vi "PH_Sixpack.set Status.vi"(0 "VI in":refnum<vi>, 2 "Status":T1, 5 "error in (no error)":errorcluster) -> (14 "VI out":refnum<vi>, 19 "error out":errorcluster)   [LabVIEW 2014, in "PH_Sixpack.lvlib"]
doc: "This VI sets the internal status."
uses:
  PH_Sixpack.lvlib
  PH_Sixpack.Status.ctl
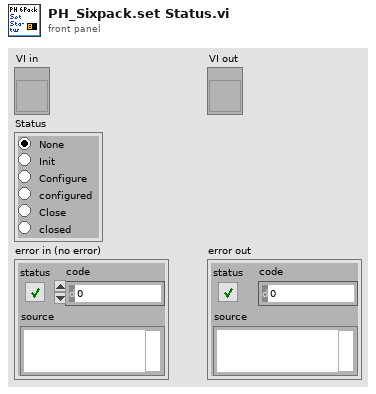
[diagram p1: front panel]
types:
  T1 = typedef "PH_Sixpack.lvlib/PH_Sixpack.Status.ctl" = enum32{"None", "Init", "Configure", "configured", "Close", "closed"}
  T2 = typedef "PH_Sixpack.lvlib/PH_Sixpack.i attribute.ctl" = cluster{"Information":cluster{"SixPack ID(0)":u16, "BaudRate(19200)":u16, "COM Port":enum32{"COM1", "COM2", "COM3", "COM4", "COM5", "COM6", "COM7", "COM8", "COM9"}, "HANDLE":i32}, "Serial Number":dbl, "Firmwareversion":dbl, "Axes":T3[], "Status":T1, "Axis to do a RefSearch":i32, "GUI Refs":cluster{"Information":refnum<vi>, "Serial Number":refnum<vi>, "Firmwareversion":refnum<vi>, "Status":refnum<vi>, "Axis to do a RefSearch":refnum<vi>, "Axes Configuration (Sixpack)":refnum<vi>, "Inputs":refnum<vi>, "PeriodicInterval [ms]":refnum<vi>}, "Constructor finished":bool, "Ignore Error":bool}
  T3 = typedef "PH_Sixpack.lvlib/PH_Sixpack.Axis Cluster.ctl" = cluster{"Config":T4, "To set?":cluster{"VmaxAmax":bool, "I max":bool, "VStartVminDivi":bool, "Ref Search Parameter":bool, "Stopswitch Limits":bool, "Axis Parameter":bool, "I Control":bool}}
  T4 = typedef "PH_Sixpack.lvlib/PH_Sixpack.Axis Configuration.ctl" = cluster{"VmaxAmax":T5, "I max (50%)":T6, "VStartVminDivi":T7, "Ref Search Parameter":T8, "Stopswitch Limits":T9, "Axis Parameter":T10, "I Control":T13}
  T5 = typedef "Sixpack - Driver.lvlib/VmaxAmax.ctl" = cluster{"VMax(511)":u16, "AMax(128)":u16}
  T6 = typedef "Sixpack - Driver.lvlib/PeakCurrent.ctl" = dbl
  T7 = typedef "Sixpack - Driver.lvlib/VStartVmin.ctl" = cluster{"VStart(5)":u16, "Vmin(4)":u16, "Div i (2)":enum8{"0", "1", "2", "3"}}
  T8 = typedef "Sixpack - Driver.lvlib/Ref Search Parameter.ctl" = cluster{"VRefMax(100)":u16, "DebouncingTime (22ms)":u8}
  T9 = typedef "Sixpack - Driver.lvlib/Stopswitch Limits.ctl" = cluster{"MinLeft(0)":u16, "MaxRight(1023)":u16}
  T10 = typedef "Sixpack - Driver.lvlib/Motor Parameter.ctl" = cluster{"Poslimit (6400)":u32, "P5 Bits":T11, "P6 Bits":T12}
  T11 = typedef "Sixpack - Driver.lvlib/MotorParameter_P5.ctl" = cluster{"MT_PI":bool, "MT_ROTARY":bool, "MT_AUTONULLCMD":bool, "MT_TESTNULL":bool, "MT_NULLLEFT":bool, "MT_NULLCENTRE":bool, "MT_STOPNULL":bool, "MT_FILTERSWITCH":bool}
  T12 = typedef "Sixpack - Driver.lvlib/MotorParameter_P6.ctl" = cluster{"MT_OPTIMIZEWAY":bool, "MT_FASTREF":bool, "MT_MECHREF":bool, "MT_DELAYTESTNULL":bool, "MT_STOPSOFT":bool, "MT_STOPNOREF":bool, "MT_NULLPOSITIVE":bool, "MUT_STOPFULSTEPS":bool}
  T13 = typedef "Sixpack - Driver.lvlib/Current Control.ctl" = cluster{"PowerDownDelay (500)":u16, "PowerDown (0%)":T14, "Standing (50%)":T14, "Running (75%)":T14, "Accelerating (100%)":T14}
  T14 = typedef "Sixpack - Driver.lvlib/Current.ctl" = enum8{"100%", "75%", "50%", "38%", "25%", "19%", "13%", "9%", "0%"}
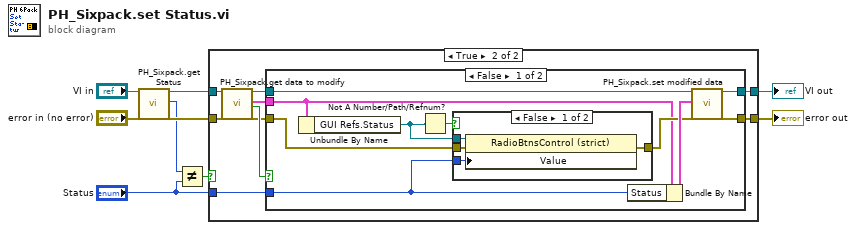
[diagram p0: block diagram]
diagram:
  n1 = call "PH_Sixpack.get Status.vi"("VI in"="VI in", "error in (no error)"="error in (no error)") -> ("VI out"=w6:refnum<vi>, "Status"=w5:T1, "error out"=w7:errorcluster)  [unwired: 14 in, 1 out]
  n2 = Not Equal?(x=w5, y="Status") -> (x != y?=w3:bool)
  n3 = case shown="True" w3 {
    tunnel: [w10 w20] -> w9
    tunnel: [w11 w19] -> w8
    tunnel: w7 -> [w10 w14]
    tunnel: w6 -> [w11 w13]
    tunnel: "Status" -> [_ w12]
    frame False {
    }
    frame True {
      n4 = call "PH_Sixpack.get data to modify.vi"("i ref in"=w13, "error in (no error)"=w14) -> ("i ref out"=w17:refnum<vi>, "i attribute"=w15:T2, "timed out"=w18:bool, "error out"=w16:errorcluster)  [unwired: 14 in]
      n5 = case shown="False" w18 {
        tunnel: w15 -> [w24 _]
        tunnel: [w29 w36] -> w20
        tunnel: w16 -> [w28 w36]
        tunnel: w17 -> [w27 w37]
        tunnel: [w26 w37] -> w19
        tunnel: w12 -> [w23 _]
        frame False {
          n6 = Unbundle By Name(w24) -> ("GUI Refs.Status"=w21:refnum<vi>)
          n7 = Not A Number/Path/Refnum?(number/path/refnum=w21) -> (NaN/Path/Refnum?=w22:bool)
          n8 = case shown="False" w22 {
            tunnel: w28 -> [w34 w35]
            tunnel: [w33 w35] -> w25
            tunnel: w21 -> [w32 _]
            tunnel: w23 -> [w31 _]
            frame False {
              n9 = property class="RadioBtnsControl (strict)"(reference=w32, error in=w34, "Value"=w31) -> (error out=w33:errorcluster)  [unwired: 1 out]
            }
            frame True {
            }
          }
          n10 = Bundle By Name(cluster=w24, "Status"=w23) -> (w30:T2)
          n11 = call "PH_Sixpack.set modified data.vi"("i ref in"=w27, "i attribute"=w30, "error in (no error)"=w25) -> ("i ref out"=w26:refnum<vi>, "error out"=w29:errorcluster)  [unwired: 15 in]
        }
        frame True {
        }
      }
    }
  }
  "error out" <- w9
  "VI out" <- w8
